vi "Configure Marker Type.vi"(0 "VISA resource name":refnum<visa-resource-name>, 1 "Enable Marker List (F:Disable)":bool, 2 "Marker Type (2:Integral Power)":i32(ring)=2 items=["Total", "Average", "Integral Power", "Power Density", "Peak Level"], 3 "Tracking (0:Off)":i32(ring) items=["Off", "On"], 5 "Marker Target (0:Marker 1)":i32(ring) items=["Marker 1", "Marker 2", "Marker 3", "Marker 4", "Marker 5", "Marker 6", "Marker 7", "Marker 8", "Marker 9", "Marker 10"], 7 "Trace (0:A)":i32(ring) items=["A", "B", "C", "D", "E", "F"], 9 "Marker Mode (1:On)":i32(ring)=1 items=["Off", "On", "Delta", "Fixed"], 11 "error in (no error)":errorcluster, 12 "Marker Reference (0:Marker 1)":i32(ring) items=["Marker 1", "Marker 2", "Marker 3", "Marker 4", "Marker 5", "Marker 6", "Marker 7", "Marker 8", "Marker 9", "Marker 10", "Active Marker"], 13 "Enable Power Marker (F:Disable)":bool) -> (4 "VISA resource name out":refnum<visa-resource-name>, 15 "error out":errorcluster)   [LabVIEW 2023, in "Anritsu Signal Analyzer Series.lvlib"]
doc: "Configures the marker type settings of the spectrum analyzer."
uses:
  Anritsu Signal Analyzer Series.lvlib
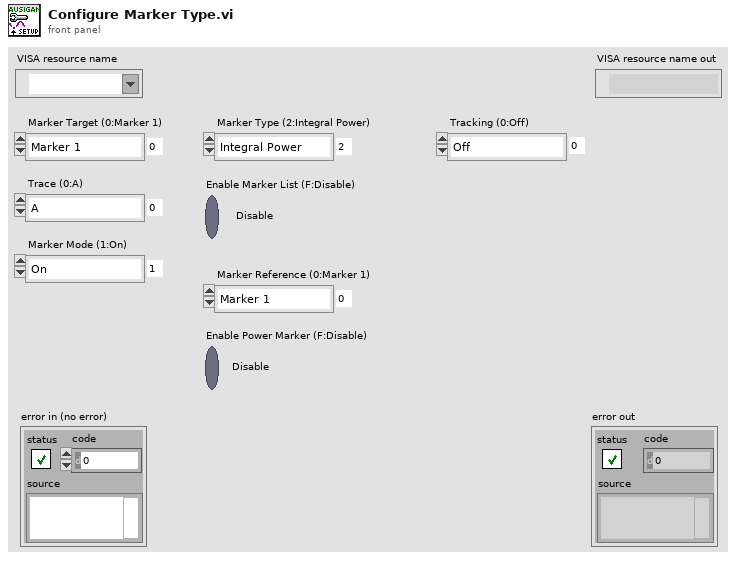
[diagram p1: front panel]
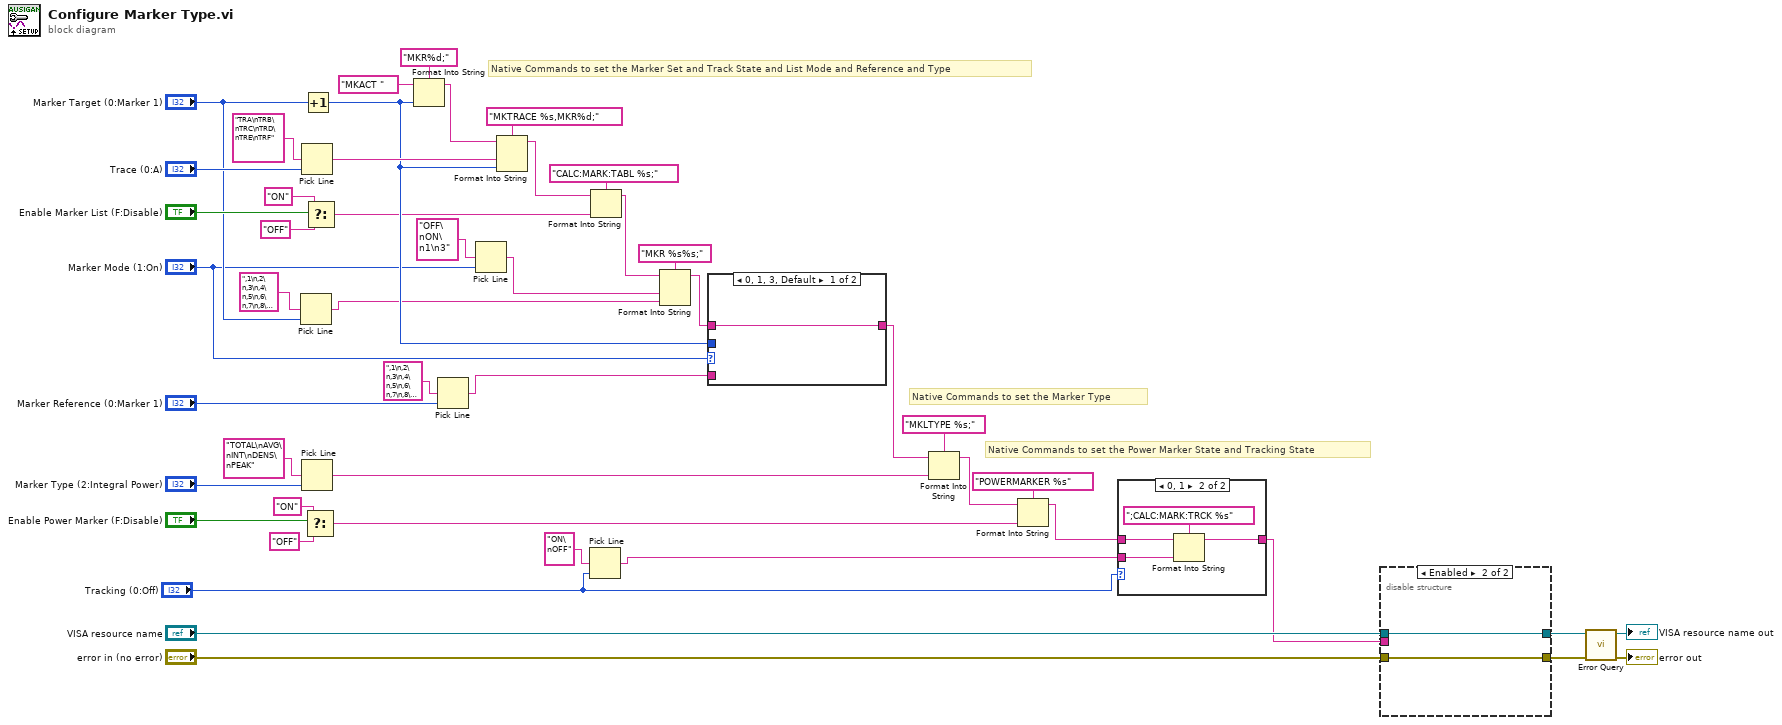
[diagram p0: block diagram]
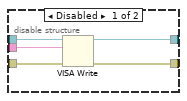
[diagram p2: hidden frame]
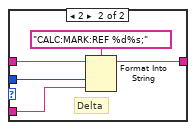
[diagram p4: hidden frame]
diagram:
  # "Native Commands to set the Marker Type"
  # "Native Commands to set the Power Marker State and Tracking State"
  # "Native Commands to set the Marker Set and Track State and List Mode and Reference and Type"
  n1 = Pick Line(multi-line string=",1\n,2\n,3\n,4\n,5\n,6\n,7\n,8\n,9\n,10" ("文字列"), line index="Marker Target (0:Marker 1)") -> (output string=w7:string)  [unwired: 1 in]
  n2 = Pick Line(multi-line string="TRA\nTRB\nTRC\nTRD\nTRE\nTRF" ("複数行文字列"), line index="Trace (0:A)") -> (output string=w26:string)  [unwired: 1 in]
  n3 = Pick Line(multi-line string="TOTAL\nAVG\nINT\nDENS\nPEAK" ("複数行文字列"), line index="Marker Type (2:Integral Power)") -> (output string=w23:string)  [unwired: 1 in]
  n4 = Increment(x="Marker Target (0:Marker 1)") -> (x+1=w25:i32)
  n5 = Select(t="ON" ("複数行文字列"), s="Enable Power Marker (F:Disable)", f="OFF" ("複数行文字列")) -> (s? t:f=w13:string)
  n6 = Select(t="ON" ("複数行文字列"), s="Enable Marker List (F:Disable)", f="OFF" ("複数行文字列")) -> (s? t:f=w15:string)
  n7 = Format Into String(format string="MKR%d;" ("_CommandSet"), initial string="MKACT ", w25) -> (resulting string=w41:string)  [unwired: 1 in, 1 out]
  n8 = Pick Line(multi-line string=",1\n,2\n,3\n,4\n,5\n,6\n,7\n,8\n,9\n,10\n" ("文字列"), line index="Marker Reference (0:Marker 1)") -> (output string=w10:string)  [unwired: 1 in]
  n9 = Pick Line(multi-line string="OFF\nON\n1\n3" ("複数行文字列"), line index="Marker Mode (1:On)") -> (output string=w4:string)  [unwired: 1 in]
  n10 = Format Into String(format string="MKTRACE %s,MKR%d;", initial string=w41, w26, w25) -> (resulting string=w39:string)  [unwired: 1 in, 1 out]
  n11 = Pick Line(multi-line string="ON\nOFF" ("複数行文字列"), line index="Tracking (0:Off)") -> (output string=w27:string)  [unwired: 1 in]
  n12 = Format Into String(format string="CALC:MARK:TABL %s;" ("_CommandSet"), initial string=w39, w15) -> (resulting string=w37:string)  [unwired: 1 in, 1 out]
  n13 = Format Into String(format string="MKR %s%s;" ("_CommandSet"), initial string=w37, w4, w7) -> (resulting string=w35:string)  [unwired: 1 in, 1 out]
  n14 = case shown="0, 1, 3, Default" "Marker Mode (1:On)" {
    tunnel: w25 -> [_ w54]
    tunnel: w10 -> [_ w53]
    tunnel: w35 -> [w49 w52]
    tunnel: [w49 w50] -> w34
    frame 0, 1, 3, Default {
    }
    frame 2 {
      # "Delta"
      n15 = Format Into String(format string="CALC:MARK:REF %d%s;" ("_CommandSet"), initial string=w52, w54, w53) -> (resulting string=w50:string)  [unwired: 1 in, 1 out]
    }
  }
  n16 = Format Into String(format string="MKLTYPE %s;" ("_CommandSet"), initial string=w34, w23) -> (resulting string=w21:string)  [unwired: 1 in, 1 out]
  n17 = Format Into String(format string="POWERMARKER %s" ("_CommandSet"), initial string=w21, w13) -> (resulting string=w3:string)  [unwired: 1 in, 1 out]
  n18 = case shown="0, 1" "Tracking (0:Off)" {
    tunnel: w27 -> [_ w59]
    tunnel: w3 -> [w55 w58]
    tunnel: [w55 w56] -> w1
    frame Default {
    }
    frame 0, 1 {
      n19 = Format Into String(format string=";CALC:MARK:TRCK %s" ("_CommandSet"), initial string=w58, w59) -> (resulting string=w56:string)  [unwired: 1 in, 1 out]
    }
  }
  n20 = disable-structure shown="Enabled" {
    disable-tunnel: "VISA resource name" -> [w64 w66]
    disable-tunnel: "error in (no error)" -> [w63 w65]
    disable-tunnel: [w62 w65] -> w32
    disable-tunnel: [w61 w66] -> w31
    disable-tunnel: w1 -> [w60 _]
    frame Disabled {
      n21 = VISA Write(VISA resource name=w64, write buffer=w60, error in (no error)=w63) -> (VISA resource name out=w61:refnum<visa-resource-name>, error out=w62:errorcluster)  [unwired: 1 out]
    }
    frame Enabled {
    }
  }
  n22 = call "Error Query.vi"("error in (no error)"=w32, "VISA resource name"=w31) -> ("error out"=→"error out":errorcluster, "VISA resource name out"=→"VISA resource name out":refnum<visa-resource-name>)  [unwired: 6 in, 2 out]
